vi "Actor Core.vi"(8 "error in":errorcluster, 11 "Measurement Setup in":refnum<class "Measurement Setup.lvclass">) -> (0 "error out":errorcluster, 3 "Actor out":refnum<class "Actor.lvclass">)   [LabVIEW 2015, in "Measurement Setup Controller.lvlib" / "Measurement Setup.lvclass"]
doc: "(<B>Filename</B>: Actor Framework.lvlib:Actor.lvclass:Actor Core.vi)\n\nReceives messages to the actor, reacts to them, and initiates any error handling that may shut the actor down.\n\nDescendant classes may override this VI to append parallel tasks for the actor to complete while it handles messages. Overrides use the Call Parent Method node."
uses:
  Measurement Setup.lvclass
  <vilib>/ActorFramework/Actor/Actor.lvclass
  <userlib>/Common Components/Controller/Controller.lvclass
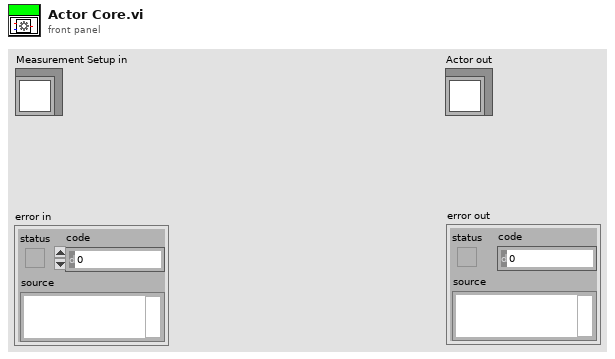
[diagram p1: front panel]
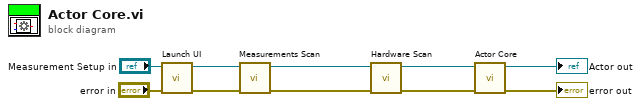
[diagram p0: block diagram]
diagram:
  n1 = call-dynamic "Launch UI.vi"("error in (no error)"="error in", "UI Controller in"="Measurement Setup in") -> ("error out"=w6:errorcluster, "UI Controller out"=w5:refnum<class "Measurement Setup.lvclass">)  [unwired: 8 in]
  n2 = call-dynamic "Measurements Scan.vi"("error in (no error)"=w6, "Controller in"=w5) -> ("error out"=w3:errorcluster, "Controller out"=w7:refnum<class "Measurement Setup.lvclass">)  [unwired: 8 in]
  n3 = call-dynamic "Hardware Scan.vi"("error in (no error)"=w3, "Controller in"=w7) -> ("error out"=w2:errorcluster, "Controller out"=w4:refnum<class "Measurement Setup.lvclass">)  [unwired: 8 in]
  n4 = call-parent "Actor Core.vi"("error in"=w2, "Actor in"=w4) -> ("error out"=→"error out":errorcluster, "Actor out"=→"Actor out":refnum<class "Actor.lvclass">)  [unwired: 8 in]
